vi "AnalogIN_Normieren_PC.vi"(7 "Analogwert":sgl, 8 "Obergrenze":sgl, 9 "Untergrenze":sgl, 10 "Max Analogwert":sgl, 11 "Min Analogwert":sgl) -> (3 "Normierter Wert":sgl)   [LabVIEW 2020, in "allgemeine Sub-VIs.lvlib"]
uses:
  allgemeine Sub-VIs.lvlib
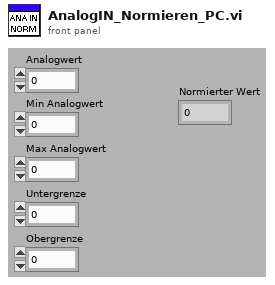
[diagram p1: front panel]
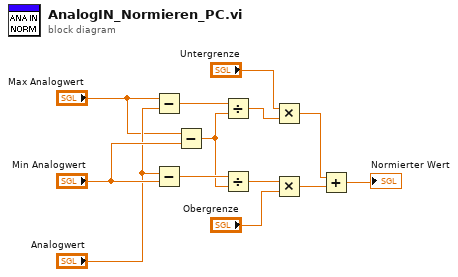
[diagram p0: block diagram]
diagram:
  n1 = Subtract(x="Max Analogwert", y="Analogwert") -> (x-y=w13:sgl)
  n2 = Subtract(x="Analogwert", y="Min Analogwert") -> (x-y=w12:sgl)
  n3 = Subtract(x="Max Analogwert", y="Min Analogwert") -> (x-y=w11:sgl)
  n4 = Divide(x=w13, y=w11) -> (x/y=w10:sgl)
  n5 = Divide(x=w12, y=w11) -> (x/y=w9:sgl)
  n6 = Multiply(x="Untergrenze", y=w10) -> (x*y=w5:sgl)
  n7 = Multiply(x=w9, y="Obergrenze") -> (x*y=w6:sgl)
  n8 = Add(x=w5, y=w6) -> (x+y=→"Normierter Wert":sgl)
